vi "Clear Path.vi"(9 "Hallway":string[](array[string]), 10 "Hallway Position":i32, 11 "Room":string) -> (3 "Clear Path?":bool)   [LabVIEW 2019, in "23.lvlib"]
uses:
  23.lvlib
  Destination Room Position.vi
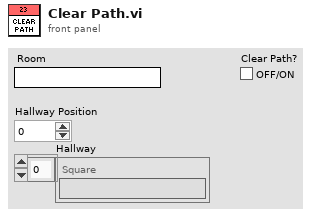
[diagram p1: front panel]
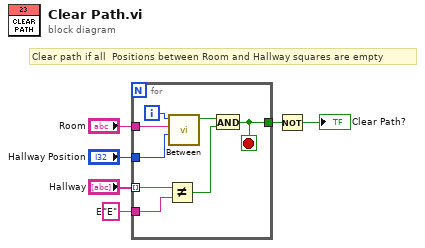
[diagram p0: block diagram]
diagram:
  w4 = "E"  # E
  # "Clear path if all  Positions between Room and Hallway squares are empty"
  n1 = for {
    tunnel: "Hallway" -> [w10] mode=indexing
    tunnel: "Hallway Position" -> [w13]
    tunnel: "Room" -> [w12]
    tunnel: w4 -> [w9]
    tunnel: [w7] -> w5
    i -> [w14]
    stop <- w7 stop-if-true
    n2 = Not Equal?(x=w10, y=w9) -> (x != y?=w8:bool)
    n3 = call "Between.vi"("Hallway Position"=w13, "Room"=w12, "Position"=w14) -> ("Betwwen?"=w11:bool)  [unwired: 8 in]
    n4 = And(x=w11, y=w8) -> (x .and. y?=w7:bool)
  }
  n5 = Not(x=w5) -> (.not. x?=→"Clear Path?":bool)
